vi "1820_IPSTime_to_TimeStamp.vi"(11 "IPS Time":string="11:11:48") -> (3 "time stamp":timestamp format="%<%I:%M:%S %p>T")   [LabVIEW 2016]
uses:
  <vilib>/Utility/miscctls.llb/LVDateTimeRec.ctl
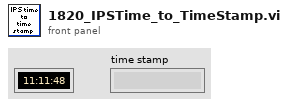
[diagram p1: front panel]
types:
  T1 = typedef "LVDateTimeRec.ctl" = cluster{"fractional second":dbl, "second":i32, "minute":i32, "hour":i32, "day of month":i32, "month":i32, "year":i32, "day of week":i32, "day of year":i32, "DST":i32}
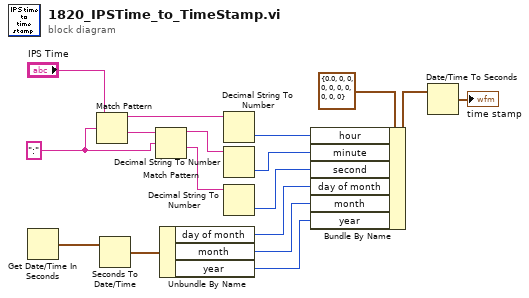
[diagram p0: block diagram]
diagram:
  w13 = ":" ("regular expression")
  n1 = Get Date/Time In Seconds() -> (seconds since 1Jan1904=w5:timestamp)
  n2 = Match Pattern(string="IPS Time", regular expression=w13) -> (before substring=w12:string, after substring=w14:string)  [unwired: 1 in, 2 out]
  n3 = Seconds To Date/Time(time stamp (now)=w5) -> (date time rec=w4:T1)  [unwired: 1 in]
  n4 = Match Pattern(string=w14, regular expression=w13) -> (before substring=w11:string, after substring=w10:string)  [unwired: 1 in, 2 out]
  n5 = Unbundle By Name(w4) -> ("day of month"=w3:i32, "month"=w2:i32, "year"=w1:i32)
  n6 = Decimal String To Number(string=w12) -> (number=w7:i32)  [unwired: 2 in, 1 out]
  n7 = Decimal String To Number(string=w11) -> (number=w8:i32)  [unwired: 2 in, 1 out]
  n8 = Decimal String To Number(string=w10) -> (number=w9:i32)  [unwired: 2 in, 1 out]
  n9 = Bundle By Name(cluster=T1 {"fractional second"=0.0, "second"=0, "minute"=0, "hour"=0, "day of month"=0, "month"=0, "year"=0, "day of week"=0, "day of year"=0, "DST"=0} ("date time rec"), "hour"=w7, "minute"=w8, "second"=w9, "day of month"=w3, "month"=w2, "year"=w1) -> (w16:T1)
  n10 = Date/Time To Seconds(2:w16) -> (0:→"time stamp":timestamp)  [unwired: 1 in]
